vi "CloseStream.vi"(0 "client handle":T2, 1 "queue in":T3, 3 "error in (no error)":errorcluster) -> (7 "remaining elements":T1(array[cluster]), 10 "error out":errorcluster)   [LabVIEW 2022 SP3]
uses:
  <vilib>/httpClient/ClientHandle.ctl
  <vilib>/httpClient/LabVIEWHTTPClient.lvlib
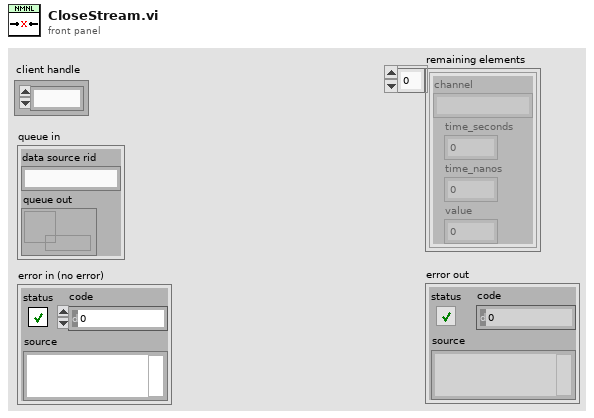
[diagram p1: front panel]
types:
  T1 = cluster{"channel":string, "time_seconds":i32, "time_nanos":i32, "value":dbl}[]
  T2 = typedef "LabVIEWHTTPClient.lvlib/ClientHandle.ctl" = refnum<k1>
  T3 = cluster{"data source rid":string, "queue out":refnum<queue>}
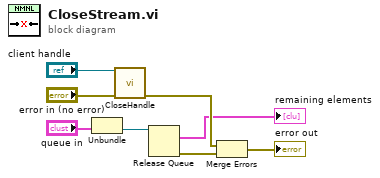
[diagram p0: block diagram]
diagram:
  n1 = Unbundle("queue in") -> ("queue out"=w5:refnum<queue>)  [unwired: 1 out]
  n2 = call <vilib>:"CloseHandle.vi"("client handle"="client handle", "error in (no error)"="error in (no error)") -> ("error out"=w3:errorcluster)  [unwired: 13 in]
  n3 = Release Queue(queue=w5) -> (remaining elements=→"remaining elements":T1, error out=w4:errorcluster)  [unwired: 2 in, 1 out]
  n4 = Merge Errors(w3, w4) -> (→"error out":errorcluster)
